vi "Function.vi"(8 "error in (no error)":errorcluster, 10 "Numeric A":T1, 11 "Two Terminal in":refnum<class "MatchPattern_STR.lvclass">) -> (0 "error out":errorcluster, 2 "Result":bool, 3 "Two Terminal out":refnum<class "MatchPattern_STR.lvclass">)   [LabVIEW 2021, in "MatchPattern_STR.lvclass"]
uses:
  MatchPattern_STR.lvclass
  Support/Compare/Two Term/STR/Support/Data Type.ctl
  MatchPattern_STR.lvclass/MatchPattern_STR.ctl
  Abs_Types/I32 Integer/Abs_I32 Integer.lvclass
  Abs_Types/String/Abs_String.lvclass
  Support/Compare/Two Term/STR/AbsComp_Two Term_STR.lvclass
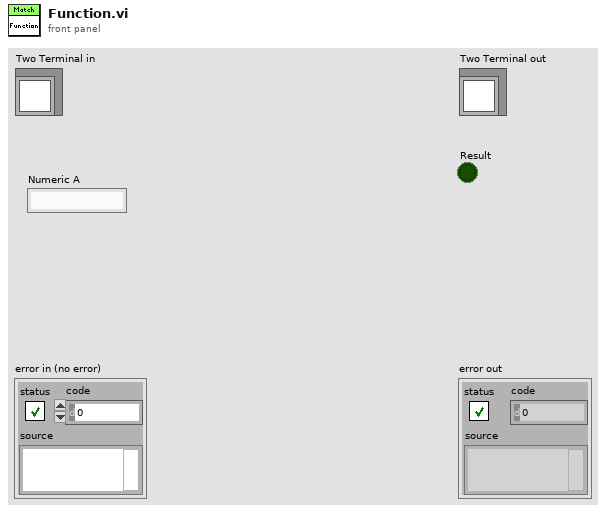
[diagram p1: front panel]
types:
  T1 = typedef "AbsComp_Two Term_STR.lvclass/Data Type.ctl" = string
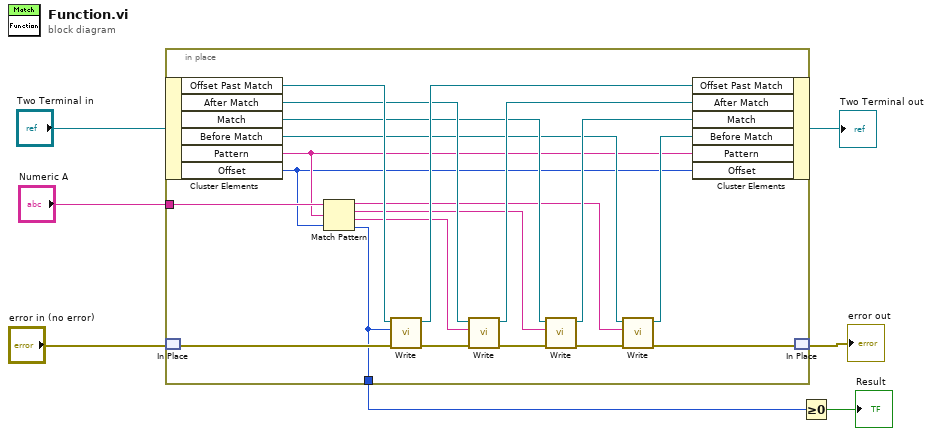
[diagram p0: block diagram]
diagram:
  n1 = in-place {
    in-place-border: "Numeric A" -> [w14]
    in-place-border: [w10] -> w1
    n2 = in-place-cluster #1("Two Terminal in") -> ("Offset Past Match"=w24:refnum<class "Abs_I32 Integer.lvclass">, "After Match"=w22:refnum<class "Abs_String.lvclass">, "Match"=w20:refnum<class "Abs_String.lvclass">, "Before Match"=w16:refnum<class "Abs_String.lvclass">, "Pattern"=w9:string, "Offset"=w8:i32)
    n3 = in-place-match #2("error in (no error)") -> (w17:errorcluster)
    n4 = Match Pattern(string=w14, regular expression=w9, offset (0)=w8) -> (before substring=w13:T1, match substring=w12:T1, after substring=w11:T1, offset past match=w10:i32)
    n5 = call-dynamic "Write.vi"("error in (no error)"=w17, "Value"=w10, "Double Float.lvclass_340760 in"=w24) -> ("error out"=w25:errorcluster, "Double Float.lvclass_340760 out"=w23:refnum<class "Abs_I32 Integer.lvclass">)  [unwired: 7 in]
    n6 = call-dynamic "Write.vi"("error in (no error)"=w25, "String"=w11, "Abs_String in"=w22) -> ("error out"=w27:errorcluster, "Abs_String out"=w21:refnum<class "Abs_String.lvclass">)  [unwired: 7 in]
    n7 = call-dynamic "Write.vi"("error in (no error)"=w27, "String"=w12, "Abs_String in"=w20) -> ("error out"=w26:errorcluster, "Abs_String out"=w19:refnum<class "Abs_String.lvclass">)  [unwired: 7 in]
    n8 = call-dynamic "Write.vi"("error in (no error)"=w26, "String"=w13, "Abs_String in"=w16) -> ("error out"=w18:errorcluster, "Abs_String out"=w15:refnum<class "Abs_String.lvclass">)  [unwired: 7 in]
    n9 = in-place-cluster #1("Offset Past Match"=w23, "After Match"=w21, "Match"=w19, "Before Match"=w15, "Pattern"=w9, "Offset"=w8) -> (→"Two Terminal out":refnum<class "MatchPattern_STR.lvclass">)
    n10 = in-place-match #2(w18) -> (→"error out":errorcluster)
  }
  n11 = Greater Or Equal To 0?(x=w1) -> (x >= 0?=→"Result":bool)
